vi "GaussianNB.vi"(8 "error in":errorcluster) -> (0 "error out":errorcluster, 3 "out":refnum<class "GaussianNB.lvclass">)   [LabVIEW 2020]
doc: "Gaussian Naive Bayes (GaussianNB)\n\n Can perform online updates to model parameters via :meth:`partial_fit`.\n For details on algorithm used to update feature means and variance online,\n see Stanford CS tech report STAN-CS-79-773 by Chan, Golub, and LeVeque:\n\n http://i.stanford.edu/pub/cstr/reports/cs/tr/79/773/CS-TR-79-773.pdf\n\n Read more in the :ref:`User Guide <gaussian_naive_bayes>`.\n\n Parameters\n ----------\n priors : array-like of shape (n_classes,)\n Prior probabilities of the classes. If specified the priors are not\n adjusted according to the data.\n\n var_smoothing : float, default=1e-9\n Portion of the largest variance of all features that is added to\n variances for calculation stability.\n\n .. versionadded:: 0.20\n\n Attributes\n ----------\n class_count_ : ndarray of shape (n_classes,)\n number of training samples observed in each class.\n\n class_prior_ : ndarray of shape (n_classes,)\n probability of each class.\n\n classes_ : ndarray of shape (n_classes,)\n class labels known to the classifier\n\n epsilon_ : float\n absolute additive value to variances\n\n sigma_ : ndarray of shape (n_classes, n_features)\n variance of each feature per class\n\n theta_ : ndarray of shape (n_classes, n_features)\n mean of each feature per class\n\n \nAvailable methods:\nFit\nPartial Fit\nPredict\nPredict Log Proba\nPredict Proba\nScore\nGet Attributes\nGet Params\nSet Params"
uses:
  GaussianNB.lvclass
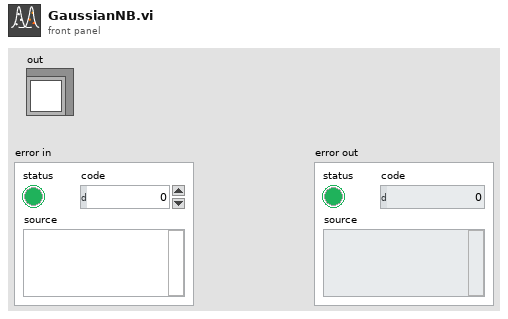
[diagram p1: front panel]
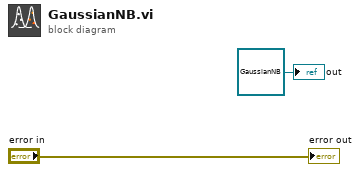
[diagram p0: block diagram]
diagram:
  "out" <- refnum<class "GaussianNB.lvclass"> refnum ("model")
  "error out" <- "error in"
